vi "Convert_Swerve_Angle.vi"(2 "Current_Position (counts)":dbl) -> (0 "Unadjusted_Counts":dbl, 1 "Angle":dbl)   [LabVIEW 2018]
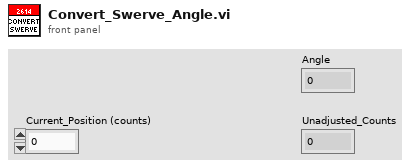
[diagram p1: front panel]
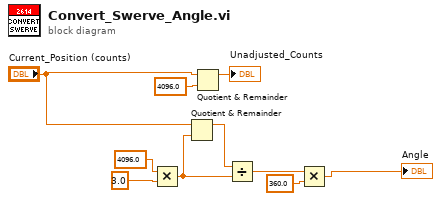
[diagram p0: block diagram]
diagram:
  n1 = Multiply(x=4096.0, y=3.0) -> (x*y=w2:dbl)
  n2 = Quotient & Remainder(x="Current_Position (counts)", y=w2) -> (x-y*floor(x/y)=w3:dbl)  [unwired: 1 out]
  n3 = Quotient & Remainder(x="Current_Position (counts)", y=4096.0) -> (x-y*floor(x/y)=→"Unadjusted_Counts":dbl)  [unwired: 1 out]
  n4 = Divide(x=w3, y=w2) -> (x/y=w8:dbl)
  n5 = Multiply(x=w8, y=360.0) -> (x*y=→"Angle":dbl)
